vi "Destroy.vi"(0 "Measurement Client Wrapper in":refnum<class "Measurement Client Wrapper.lvclass">, 11 "error in":errorcluster) -> (4 "Measurement Client Wrapper out":refnum<class "Measurement Client Wrapper.lvclass">, 15 "error out":errorcluster)   [LabVIEW 2020, in "Measurement Client Wrapper.lvclass"]
uses:
  Measurement Client Wrapper.lvclass
  Measurement Client Wrapper.lvclass/Measurement Client Wrapper.ctl
  Measurement_lv_client/Measurement_lv_client Class/Measurement_lv_client.lvclass
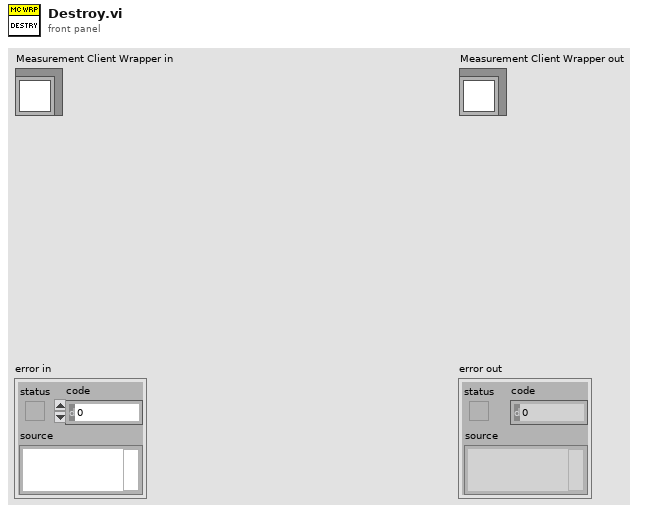
[diagram p1: front panel]
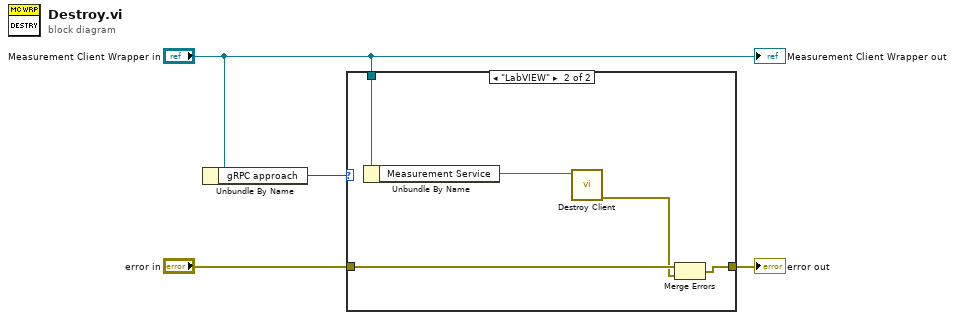
[diagram p0: block diagram]
diagram:
  n1 = Unbundle By Name("Measurement Client Wrapper in") -> ("gRPC approach"=w1:enum16{".NET", "LabVIEW"})
  n2 = case shown="\"LabVIEW\"" w1 {
    tunnel: "error in" -> [w5 w7]
    tunnel: [w5 w8] -> w3
    tunnel: "Measurement Client Wrapper in" -> [_ w10]
    frame ".NET", Default {
    }
    frame "LabVIEW" {
      n3 = Unbundle By Name(w10) -> ("Measurement Service"=w9:refnum<class "Measurement_lv_client.lvclass">)
      n4 = call "Destroy Client.vi"("gRPC Client in"=w9) -> ("error out"=w6:errorcluster)  [unwired: 9 in, 1 out]
      n5 = Merge Errors(w7, w6) -> (w8:errorcluster)
    }
  }
  "error out" <- w3
  "Measurement Client Wrapper out" <- "Measurement Client Wrapper in"
